vi "Event-Driven State Machine - Load Configuration.vi"() -> ()   [LabVIEW 2020]
uses:
  support/States.ctl
  support/State Machine Data.ctl
  support/Hardware Settings.ctl
  <vilib>/DAQmx/read.llb/DAQmx Read (Analog 2D DBL NChan NSamp).vi
  <vilib>/DAQmx/write.llb/DAQmx Write (Analog DBL 1Chan 1Samp).vi
  <vilib>/DAQmx/create/channels.llb/DAQmx Create Channel (AI-Voltage-Basic).vi
  <vilib>/DAQmx/configure/timing.llb/DAQmx Timing (Sample Clock).vi
  <vilib>/DAQmx/miscellaneous.llb/DAQmx Fill In Error Info.vi
  <vilib>/Utility/file.llb/Write Delimited Spreadsheet (DBL).vi
  <vilib>/DAQmx/create/channels.llb/DAQmx Create Channel (AO-Voltage-Basic).vi
panel:
  in  "Generate Stimulus":bool
  out "RMS Results Per Channel":dbl[](array[numeric])
  out "Threshold exceeded?":bool
  in  "Acquire":bool
  in  "Threshold (rms)":dbl=1.0
  in  "Clear":bool
  in  "Exit":bool
  out "Graph":dbl[][](graph)
  # "Analysis"
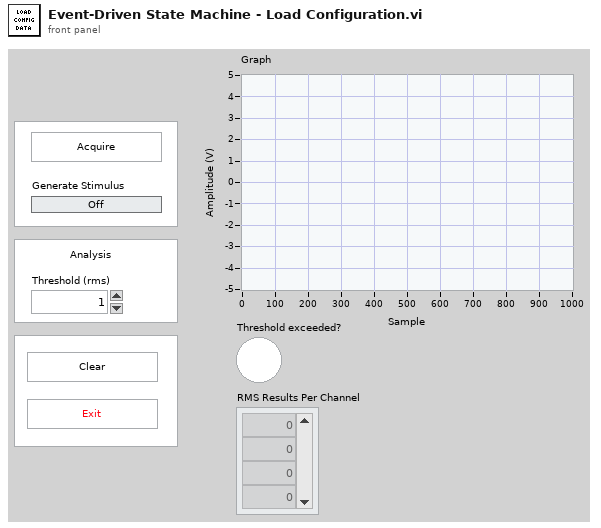
[diagram p1: front panel]
types:
  T1 = typedef "Hardware Settings.ctl" = cluster{"AI Voltage Channel":tag, "Sample Rate (Hz)":dbl, "Samples per channel":i32, "AO Voltage Channel":tag}
  T2 = typedef "State Machine Data.ctl" = cluster{"Acquisition Data":dbl[][], "Stimulus Value":bool}
  T3 = typedef "States.ctl" = enum16{"Initialize", "Wait for Event", "Acquire", "Analyze", "Log", "Clear", "Update Graph", "Update Stumulus", "Exit"}
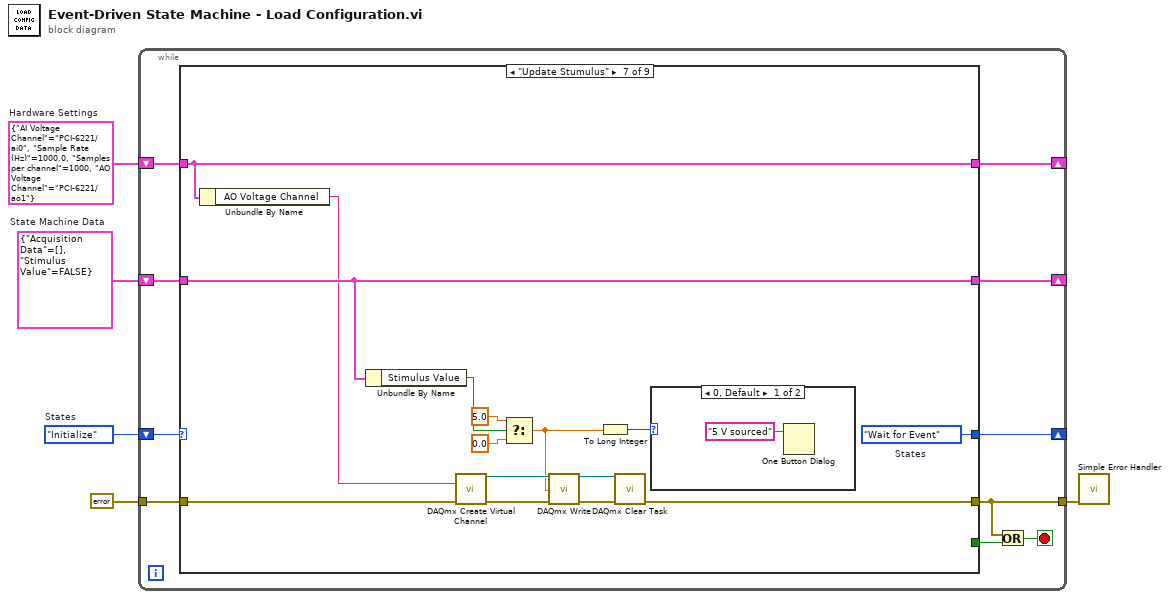
[diagram p0: block diagram]
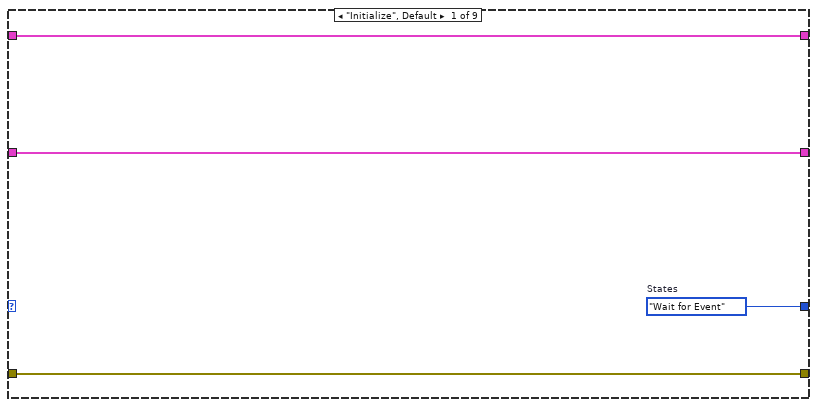
[diagram p2: hidden frame]
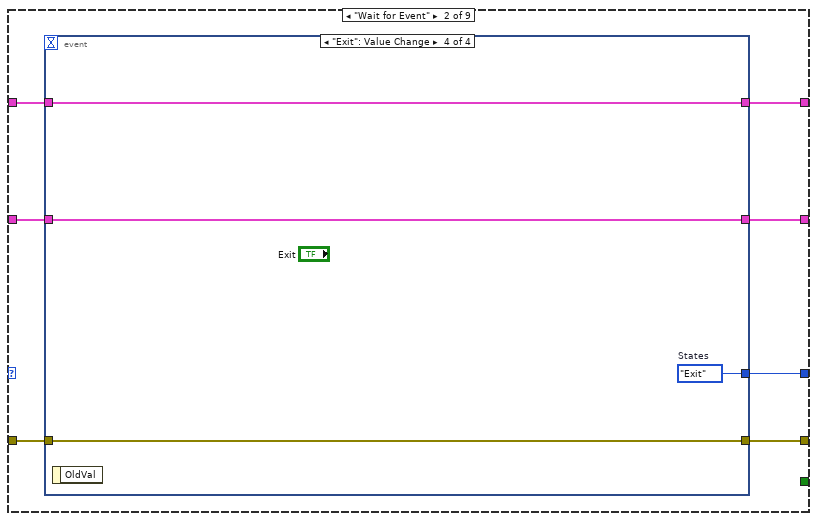
[diagram p3: hidden frame]
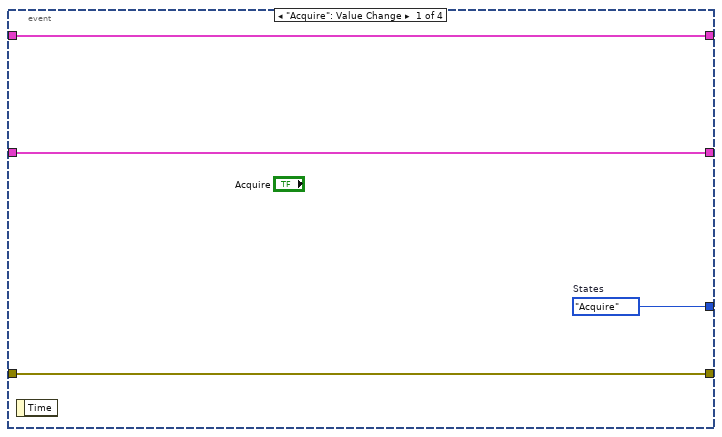
[diagram p4: hidden frame]
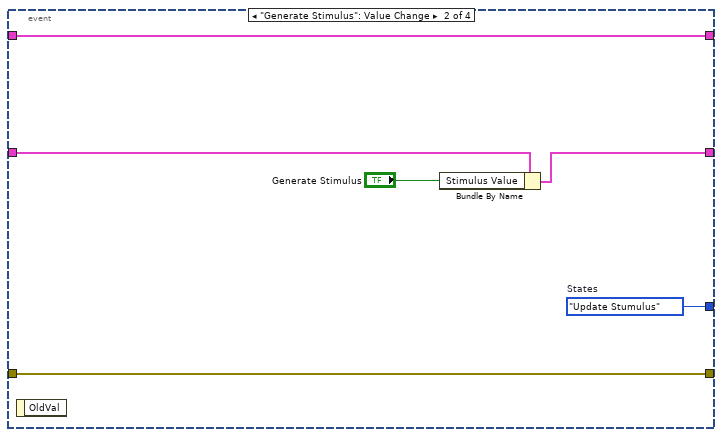
[diagram p5: hidden frame]
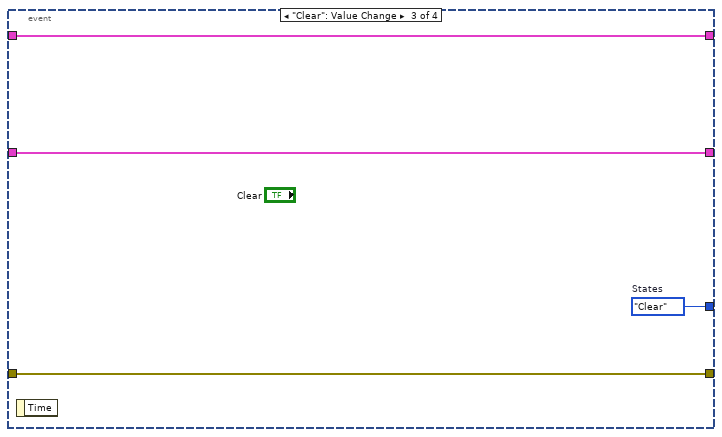
[diagram p6: hidden frame]
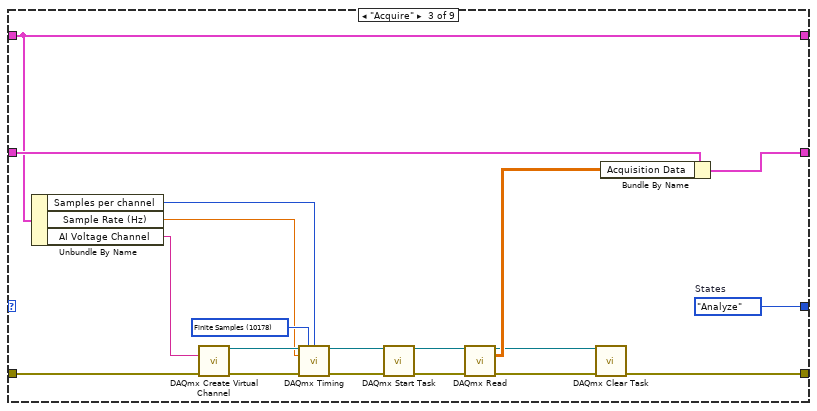
[diagram p7: hidden frame]
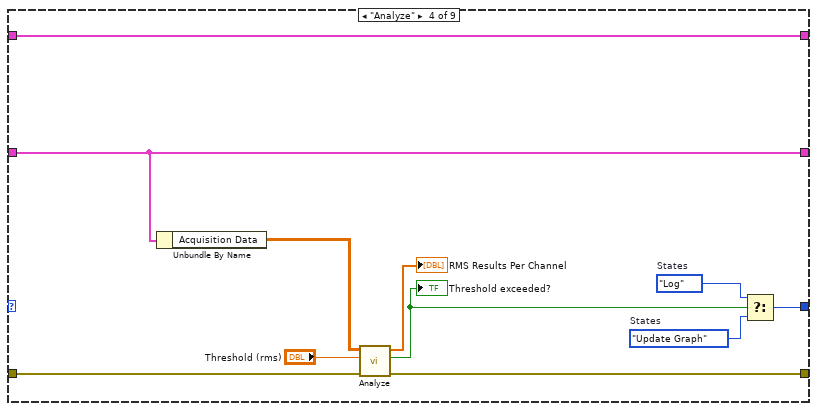
[diagram p8: hidden frame]
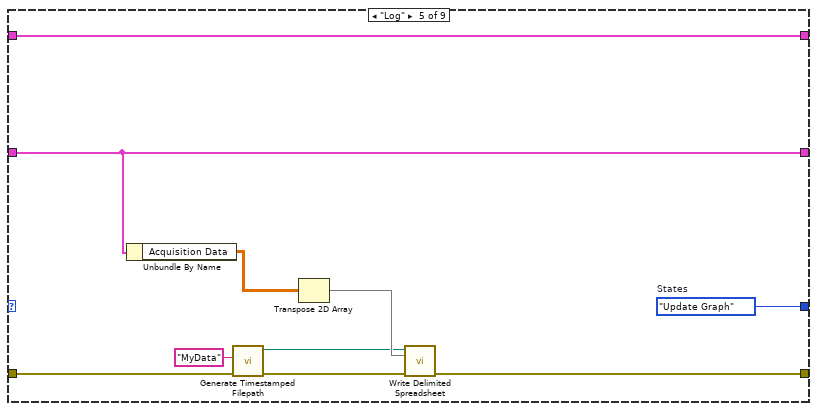
[diagram p9: hidden frame]
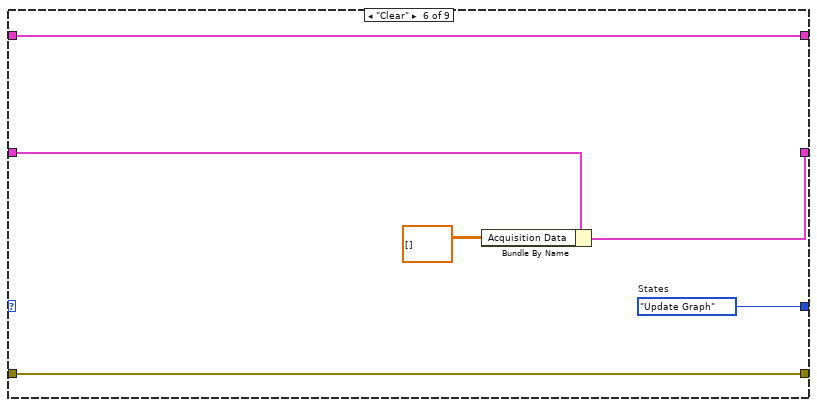
[diagram p10: hidden frame]
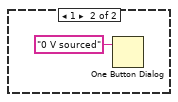
[diagram p11: hidden frame]
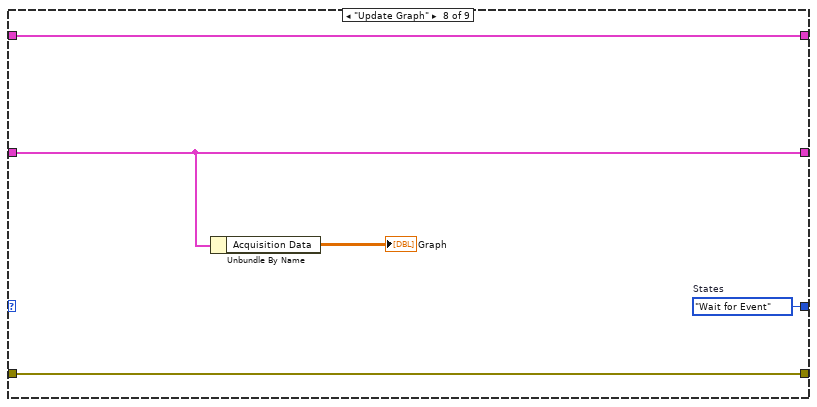
[diagram p12: hidden frame]
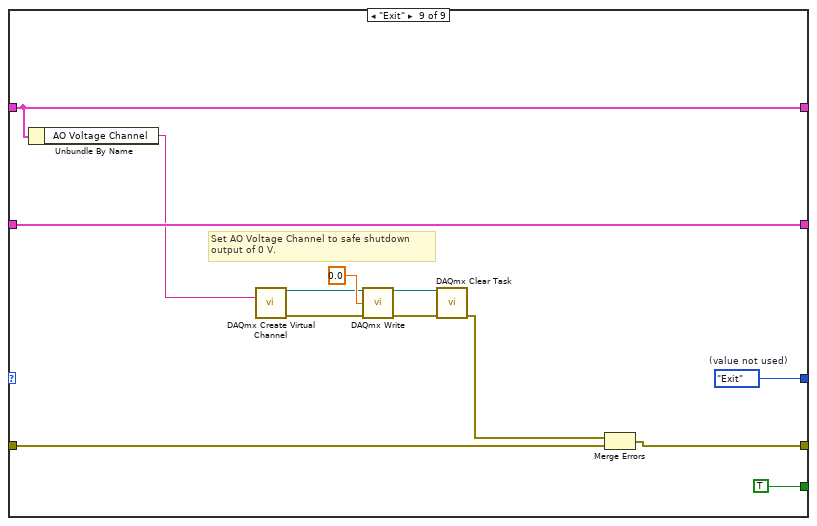
[diagram p13: hidden frame]
diagram:
  w2 = T1 {"AI Voltage Channel"="PCI-6221/ai0", "Sample Rate (Hz)"=1000.0, "Samples per channel"=1000, "AO Voltage Channel"="PCI-6221/ao1"}  # Hardware Settings
  w5 = T2 {"Acquisition Data"=[], "Stimulus Value"=FALSE}  # State Machine Data
  w4 = States."Initialize"  # States
  n1 = while {
    tunnel: errorcluster {"status"=FALSE, "code"=0, "source"=""} ("error constant") -> [w14]
    tunnel: [w10] -> w1
    shift-right: [w12] -> _
    shift-left: w5 -> [w13]
    shift-right: [w11] -> _
    shift-left: w4 -> [w15]
    shift-right: [w6] -> _
    shift-left: w2 -> [w7]
    stop <- w9 stop-if-true
    n2 = case shown="\"Update Stumulus\"" w15 {
      tunnel: w14 -> [w19 w24 w63 w73 w83 w90 w94 w111 w114]
      tunnel: [w19 w23 w58 w72 w77 w90 w93 w111 w113] -> w10
      tunnel: [w18 w25 w55 w74 w84 w88 w105 w112 w125] -> w12
      tunnel: w13 -> [w18 w26 w56 w74 w84 w89 w105 w112 w125]
      tunnel: [w17 w22 w57 w68 w76 w86 w95 w110 w123] -> w11
      tunnel: [_ _ _ _ _ _ _ _ TRUE] -> w8
      tunnel: w7 -> [w16 w21 w48 w64 w75 w85 w91 w108 w122]
      tunnel: [w16 w20 w48 w64 w75 w85 w91 w108 w122] -> w6
      frame "Initialize", Default {
        w17 = States."Wait for Event"  # States
      }
      frame "Wait for Event" {
        n3 = event shown="[3] \"Exit\": Value Change" {
          selector: _ -> [_ _ _ _]
          dyn-events: _ -> [_ _ _ _]
          timeout: _ -> [_ _ _ _]
          tunnel: w26 -> [w30 w36 w40 w43]
          tunnel: [w30 w35 w40 w43] -> w25
          tunnel: w24 -> [w29 w32 w39 w44]
          tunnel: [w29 w32 w39 w44] -> w23
          tunnel: [w28 w33 w38 w42] -> w22
          tunnel: w21 -> [w27 w31 w37 w41]
          tunnel: [w27 w31 w37 w41] -> w20
          event "Acquire": Value Change {
            w28 = States."Acquire"  # States
            n4 = event-data() -> ()  [unwired: 1 in, 1 out]
          }
          event "Generate Stimulus": Value Change {
            w33 = States."Update Stumulus"  # States
            n5 = event-data() -> ()  [unwired: 1 in, 1 out]
            n6 = Bundle By Name(cluster=w36, "Stimulus Value"="Generate Stimulus") -> (w35:T2)
          }
          event "Clear": Value Change {
            w38 = States."Clear"  # States
            n7 = event-data() -> ()  [unwired: 1 in, 1 out]
          }
          event "Exit": Value Change {
            w42 = States."Exit"  # States
            n8 = event-data() -> ()  [unwired: 1 in, 1 out]
          }
        }
      }
      frame "Acquire" {
        w54 = 10178 items=["Finite Samples"=10178, "Continuous Samples"=10123, "Hardware Timed Single Point"=12522] ("sample mode")
        w57 = States."Analyze"  # States
        n9 = Unbundle By Name(w48) -> ("Samples per channel"=w45:i32, "Sample Rate (Hz)"=w46:dbl, "AI Voltage Channel"=w47:tag)
        n10 = call-poly <vilib>:"DAQmx Create Virtual Channel.vi"("physical channels"=w47, "error in"=w63) -> ("task out"=w52:refnum<k21>, "error out"=w62:errorcluster)  [unwired: 12 in]
        n11 = call-poly <vilib>:"DAQmx Timing.vi"("task/channels in"=w52, "sample mode"=w54, "samples per channel"=w45, "rate"=w46, "error in"=w62) -> ("task out"=w51:refnum<k21>, "error out"=w61:errorcluster)  [unwired: 9 in]
        n12 = call <vilib>:"DAQmx Start Task.vi"("task/channels in"=w51, "error in"=w61) -> ("task out"=w50:refnum<k21>, "error out"=w60:errorcluster)  [unwired: 12 in]
        n13 = call-poly <vilib>:"DAQmx Read.vi"("task/channels in"=w50, "error in"=w60) -> ("task out"=w49:refnum<k21>, "data"=w53:dbl[][], "error out"=w59:errorcluster)  [unwired: 11 in]
        n14 = call <vilib>:"DAQmx Clear Task.vi"("task in"=w49, "error in"=w59) -> ("error out"=w58:errorcluster)  [unwired: 13 in]
        n15 = Bundle By Name(cluster=w56, "Acquisition Data"=w53) -> (w55:T2)
      }
      frame "Analyze" {
        w69 = States."Update Graph"  # States
        w70 = States."Log"  # States
        n16 = Unbundle By Name(w74) -> ("Acquisition Data"=w71:dbl[][])
        n17 = call "Analyze.vi"("Error In"=w73, "Treshold (rms)"="Threshold (rms)", "N-Channel Data (2D DBL)"=w71) -> ("Error Out"=w72:errorcluster, "Threshold exceeded?"=w65:bool, "N-Channel Data RMS Results"=→"RMS Results Per Channel":dbl[])  [unwired: 5 in, 1 out]
        "Threshold exceeded?" <- w65
        n18 = Select(t=w70, s=w65, f=w69) -> (s? t:f=w68:T3)
      }
      frame "Log" {
        w76 = States."Update Graph"  # States
        n19 = Unbundle By Name(w84) -> ("Acquisition Data"=w81:dbl[][])
        n20 = call "Generate Timestamped Filepath.vi"("Error In"=w83, "appended filename"="MyData") -> ("Error Out"=w78:errorcluster, "timestamped relative filepath"=w79:path)  [unwired: 8 in]
        n21 = Transpose 2D Array(2D array=w81) -> (transposed array=w80:dbl[][])
        n22 = call-poly <vilib>:"Write Delimited Spreadsheet.vi"("file path (dialog if empty)"=w79, "2D data"=w80, "error in (no error)"=w78) -> ("error out"=w77:errorcluster)  [unwired: 11 in, 1 out]
      }
      frame "Clear" {
        w86 = States."Update Graph"  # States
        n23 = Bundle By Name(cluster=w89, "Acquisition Data"=dbl[][] []) -> (w88:T2)
      }
      frame "Update Stumulus" {
        w95 = States."Wait for Event"  # States
        n24 = Unbundle By Name(w91) -> ("AO Voltage Channel"=w92:tag)
        n25 = Unbundle By Name(w105) -> ("Stimulus Value"=w96:bool)
        n26 = call-poly <vilib>:"DAQmx Create Virtual Channel.vi"("physical channels"=w92, "error in"=w94) -> ("task out"=w102:refnum<k21>, "error out"=w101:errorcluster)  [unwired: 12 in]
        n27 = Select(t=5.0, s=w96, f=0.0) -> (s? t:f=w98:dbl)
        n28 = call-poly <vilib>:"DAQmx Write.vi"("task/channels in"=w102, "data"=w98, "error in"=w101) -> ("task out"=w100:refnum<k21>, "error out"=w99:errorcluster)  [unwired: 10 in, 1 out]
        n29 = To Long Integer(number=w98) -> (32bit integer=w97:i32)
        n30 = call <vilib>:"DAQmx Clear Task.vi"("task in"=w100, "error in"=w99) -> ("error out"=w93:errorcluster)  [unwired: 13 in]
        n31 = case shown="0, Default" w97 {
          frame 0, Default {
            n32 = One Button Dialog(message="5 V sourced") -> ()  [unwired: 1 in, 1 out]
          }
          frame 1 {
            n33 = One Button Dialog(message="0 V sourced") -> ()  [unwired: 1 in, 1 out]
          }
        }
      }
      frame "Update Graph" {
        w110 = States."Wait for Event"  # States
        n34 = Unbundle By Name(w112) -> ("Acquisition Data"=→"Graph":dbl[][])
      }
      frame "Exit" {
        w123 = States."Exit"  # (value not used)
        # "Set AO Voltage Channel to safe shutdown output of 0 V."
        n35 = Unbundle By Name(w122) -> ("AO Voltage Channel"=w121:tag)
        n36 = call-poly <vilib>:"DAQmx Create Virtual Channel.vi"("physical channels"=w121) -> ("task out"=w119:refnum<k21>, "error out"=w118:errorcluster)  [unwired: 13 in]
        n37 = call-poly <vilib>:"DAQmx Write.vi"("task/channels in"=w119, "data"=0.0, "error in"=w118) -> ("task out"=w116:refnum<k21>, "error out"=w117:errorcluster)  [unwired: 10 in, 1 out]
        n38 = call <vilib>:"DAQmx Clear Task.vi"("task in"=w116, "error in"=w117) -> ("error out"=w115:errorcluster)  [unwired: 13 in]
        n39 = Merge Errors(w115, w114) -> (w113:errorcluster)
      }
    }
    n40 = Or(x=w10, y=w8) -> (x .or. y?=w9:bool)
  }
  n41 = call <vilib>:"Simple Error Handler.vi"("error in (no error)"=w1) -> ()  [unwired: 4 in, 5 out]
